vi "STA - Wave V5 Host_Wait.vi"() -> ()   [LabVIEW 2015]
doc: "The continuous acquisition mode tells the FPGA to acquire points indefinitely until a stop command is issued or until an error is encountered (FIFO overflow, module underflow, and so on). \n\nIn this acquisition mode, explicitly call the appropriate rwfm_ConfigTiming VI and set the host application's data buffer to be many times larger than the read size. The examples use a 10X size by default. If the host application's data buffer fills, then the FPGA experiences a FIFO overflow causing the acquisition to stop."
uses:
  <vilib>/rvi/interface/nirviCloseFPGA/nirviCloseFPGA.xnode
  <vilib>/FPGAPlugInAG/Dynamic/niLvFpga_Close_Dynamic.vi
  <vilib>/NI/cRIO Wfm/cRIO Wfm.lvlib
  <vilib>/rvi/interface/nirviMethod/nirviMethod.xnode
  <vilib>/rvi/interface/nirviMethod/StockFPGA_InlinedMethodWaitForSingleIRQ.vi
  <vilib>/FPGAPlugInAG/Dynamic/niLvFpga_WaitOnIrq_Dynamic.vi
  <vilib>/rvi/interface/nirviOpenFPGA/nirviOpenFPGA.xnode
  C:/Program Files (x86)/National Instruments/LabVIEW 2015/ProjectTemplates/Source/cRIOWfm/FPGA/[FPGA] SAR Acq Main.vi
  D/Documents/LabVIEW Data/STA - Waveform V0/FPGA Bitfiles/SARAcqMain_9074.lvbitx
  FPGA Bitfiles/STA-WaveformV6_FPGATarget2_[FPGA]DeltaSigMa_HoNCM4Xd4J8.lvbitx
  FPGA/[FPGA] DeltaSig Main V6_5Mod.vi
  <vilib>/FPGAPlugInAG/cRIO-9112/niLvFpga_Open_cRIO-9112.vi
  <vilib>/rvi/interface/common/dynamic/niFpgaDynamicAddResources.vi
  <vilib>/NI/cRIO Wfm/AcqRead(InterleavedSGLs).vi
  <vilib>/LabVIEW Targets/FPGA/cRIO/shared/nicrio_ModuleControls/nicrio_cRIO-9234_ConfigModeRing.ctl
panel:
  out "error schleife":errorcluster
  out "Time Measure":dbl
  out "data rate (S/s)":u32
  out "Channel Config":T2(array[cluster]) {"Input Configuration" items=["AC Coupled", "DC Coupled", "IEPE AC Coupled"]}
  in  "Samples per Read":i32
  out "file path":path
  out "error out":errorcluster
  in  "stop":bool
  out "Waveform Graph":waveform(sgl)[](graph)
  out "Buffer Backlog":dbl caption="RT Buffer Backlog [%]" format="%#.2g"
  # "Sampling Info"
  # "Channel Info"
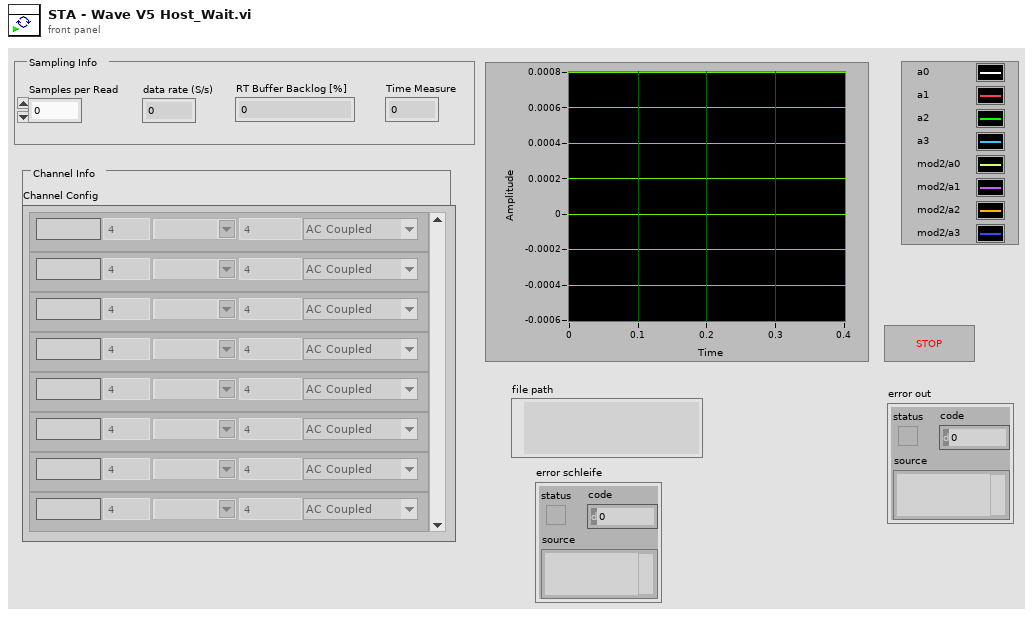
[diagram p1: front panel]
types:
  T1 = typedef "nicrio_cRIO-9234_ConfigModeRing.ctl" = u8
  T2 = cluster{"Channel Name":string, "Sensitivity mV_EU":dbl, "EU":string, "Input Configuration":T1, "dB Ref EU":dbl}[]
  T3 = enum16{"open", "open or create", "create or replace", "create", "open (read-only)"}
  T4 = typedef "Acquisition and Logging Configuration_Waveform.ctl" = cluster{"Data Rate":T5, "Samples per Read":i32, "Number of Reads to Save":i32, "Data File Name":string, "TDMS Properties":T6[], "Number of Channels":i32, "Trigger - RMS Value":dbl, "Trigger - Channel":i32, "Trigger - Time (Minute)":i32, "Channel Config":cluster{"Channel Name":string, "Sensitivity mV_EU":dbl, "EU":string, "Input Configuration":T1, "dB Ref EU":dbl}[], "data rate (S/s)":u32, "Time Measure":dbl}
  T5 = typedef "nicrio_cRIO-9234_DataRatesRing2.ctl" = u8
  T6 = typedef "TDMS Properties.ctl" = cluster{"Name":string, "Value":string}
  T7 = typedef "cRIO Wfm.lvlib/SamplingInfo.ctl" = cluster{"Number of Channels":i32, "Actual Samp Rate":dbl, "Chan Name Array":string[], "EU Chan Array":string[], "dB Ref Chan Array":dbl[]}
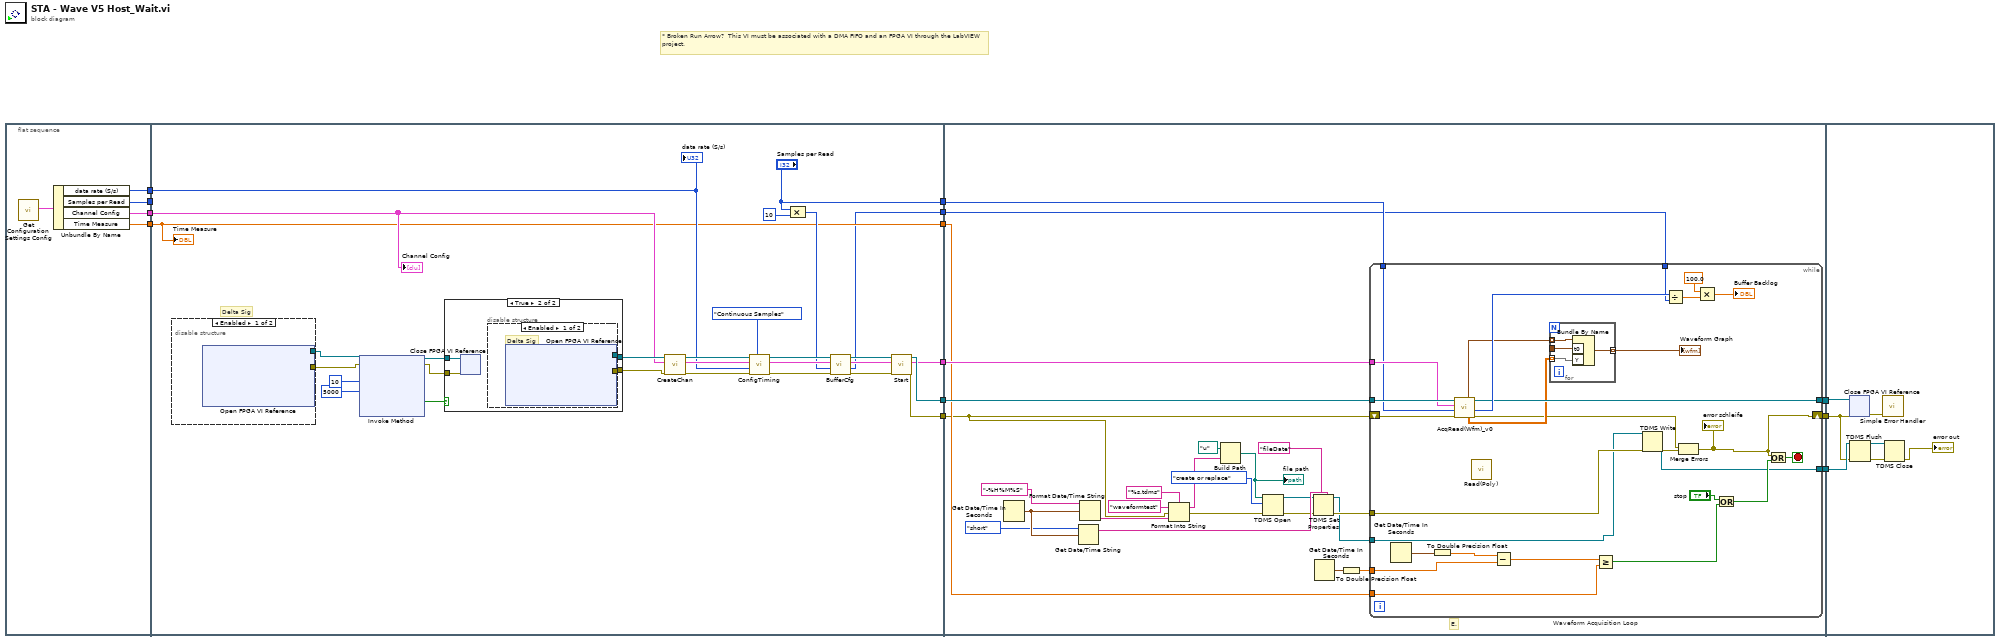
[diagram p0: block diagram]
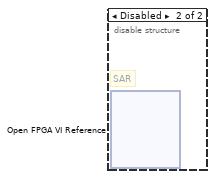
[diagram p2: hidden frame]
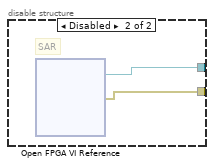
[diagram p4: hidden frame]
diagram:
  # "* Broken Run Arrow?  This VI must be associated with a DMA FIFO and an FPGA VI through the LabVIEW project."
  n1 = flat-sequence {
    tunnel: [w17] -> w13
    tunnel: [w16] -> w12
    tunnel: [w15] -> w11
    tunnel: [w14] -> w10
    tunnel: w13 -> [w28]
    tunnel: w12 -> [_]
    tunnel: w11 -> [w27]
    tunnel: w10 -> [w20]
    tunnel: ["Samples per Read"] -> w9
    tunnel: [w20] -> w8
    tunnel: [w24] -> w7
    tunnel: [w23] -> w6
    tunnel: [w22] -> w5
    tunnel: [w19] -> w4
    tunnel: w9 -> [w64]
    tunnel: w8 -> [w66]
    tunnel: w7 -> [w68]
    tunnel: w6 -> [w67]
    tunnel: w5 -> [w62]
    tunnel: w4 -> [w63]
    tunnel: [w71] -> w3
    tunnel: [w70] -> w2
    tunnel: [w69] -> w1
    tunnel: w3 -> [w125]
    tunnel: w2 -> [w123]
    tunnel: w1 -> [w124]
    frame #0 {
      n2 = call "Get Configuration Settings Config.vi"() -> ("Configuration"=w18:T4)  [unwired: 10 in, 1 out]
      n3 = Unbundle By Name(w18) -> ("data rate (S/s)"=w17:u32, "Samples per Read"=w16:i32, "Channel Config"=w15:T2, "Time Measure"=w14:dbl)
    }
    frame #1 {
      # "Delta Sig"
      n4 = disable-structure shown="Enabled" {
        disable-tunnel: [w49 _] -> w26
        disable-tunnel: [w48 _] -> w25
        frame Enabled {
          n5 = xnode "Open FPGA VI Reference"() -> ("FPGA VI Reference Out"=w49:refnum<k20>, "error out"=w48:errorcluster)  [unwired: 2 in]
        }
        frame Disabled {
          # "SAR"
          n6 = xnode "Open FPGA VI Reference"() -> ("FPGA VI Reference Out"=w51:refnum<k20>, "error out"=w50:errorcluster)  [unwired: 2 in]
        }
      }
      n7 = xnode "Invoke Method"("FPGA VI Reference In"=w26, "error in"=w25, "IRQ Number(s)"=10, "Timeout (ms)"=5000) -> ("FPGA VI Reference Out"=w44:refnum<k20>, "error out"=w45:errorcluster, "Timed Out"=w43:bool)  [unwired: 1 out]
      n8 = case shown="True" w43 {
        tunnel: w44 -> [w53 w57]
        tunnel: w45 -> [w52 w56]
        tunnel: [w53 w55] -> w47
        tunnel: [w52 w54] -> w46
        frame False {
        }
        frame True {
          n9 = xnode "Close FPGA VI Reference"("FPGA VI Reference In"=w57, "error in"=w56) -> ()  [unwired: 1 out]
          n10 = disable-structure shown="Enabled" {
            disable-tunnel: [w59 w61] -> w55
            disable-tunnel: [w58 w60] -> w54
            frame Enabled {
              # "Delta Sig"
              n11 = xnode "Open FPGA VI Reference"() -> ("FPGA VI Reference Out"=w59:refnum<k20>, "error out"=w58:errorcluster)  [unwired: 2 in]
            }
            frame Disabled {
              # "SAR"
              n12 = xnode "Open FPGA VI Reference"() -> ("FPGA VI Reference Out"=w61:refnum<k20>, "error out"=w60:errorcluster)  [unwired: 2 in]
            }
          }
        }
      }
      n13 = call <vilib>:"CreateChan.vi"("Dynamic FPGA Ref"=w47, "Channel Config"=w27, "error in"=w46) -> ("Dynamic FPGA Ref Out"=w34:refnum<k20>, "Sampling Info"=w35:T7, "error out"=w39:errorcluster)  [unwired: 5 in]
      n14 = call <vilib>:"ConfigTiming.vi"("Sample Mode"=enum16{"Finite Samples", "Continuous Samples"}."Continuous Samples", "error in"=w39, "Sample Rate"=w28, "Sampling Info In"=w35, "Dynamic FPGA Ref"=w34) -> ("error out"=w38:errorcluster, "Sampling Info Out"=w37:T7, "Dynamic FPGA Ref Out"=w36:refnum<k20>)  [unwired: 3 in, 1 out]
      n15 = Compound Arithmetic op=MULTIPLY("Samples per Read", 10 ("value")) -> (w32:i32)
      n16 = call <vilib>:"BufferCfg.vi"("error in"=w38, "Buffer Size [Samps per Chan]"=w32, "Sampling Info In"=w37, "Dynamic FPGA Ref"=w36) -> ("error out"=w31:errorcluster, "Buffer Size [Total Samples]"=w19:u32, "Sampling Info Out"=w33:T7, "Dynamic FPGA Ref Out"=w30:refnum<k20>)  [unwired: 4 out]
      n17 = call <vilib>:"Start.vi"("error in"=w31, "Sampling Info In"=w33, "Dynamic FPGA Ref"=w30) -> ("error out"=w22:errorcluster, "Sampling Info Out"=w23:T7, "Dynamic FPGA Ref Out"=w24:refnum<k20>)  [unwired: 6 out]
      "Channel Config" <- w27
      "data rate (S/s)" <- w28
      "Time Measure" <- w20
    }
    frame #2 {
      # "E."
      n18 = Get Date/Time In Seconds() -> (seconds since 1Jan1904=w86:timestamp)
      n19 = Get Date/Time String(date format (0)=enum16{"short", "long", "abbreviated"}."short", seconds (now)=w86) -> (date string=w89:string)  [unwired: 1 in, 1 out]
      n20 = Format Date/Time String(time format string (%c)="-%H%M%S", seconds (now)=w86) -> (date/time string=w76:string)  [unwired: 1 in]
      n21 = Format Into String(format string="%s.tdms", initial string="waveformtest", error in=w62, w76) -> (resulting string=w72:string, error out=w83:errorcluster)
      n22 = Build Path(base path=path "u:/", name or relative path=w72) -> (appended path=w80:path)
      "file path" <- w80
      n23 = TDMS Open(8:w83, 10:T3."create or replace" ("operation (0:open)"), 11:w80) -> (0:w78:errorcluster, 3:w79:refnum<k34>)  [unwired: 4 in]
      n24 = TDMS Set Properties(5:w89, 7:"fileDate" ("property names"), 8:w78, 11:w79) -> (0:w85:errorcluster, 3:w84:refnum<k34>)  [unwired: 2 in, 2 out]
      n25 = Get Date/Time In Seconds() -> (seconds since 1Jan1904=w88:timestamp)
      n26 = To Double Precision Float(number=w88) -> (double precision float=w87:dbl)
      n27 = while "Waveform Acquisition Loop" {
        tunnel: [w112] -> w71
        shift-right: [w90] -> w70
        shift-left: w62 -> [w118]
        tunnel: w84 -> [w94]
        tunnel: w85 -> [w95]
        tunnel: [w93] -> w69
        tunnel: w87 -> [w101]
        tunnel: w66 -> [w100]
        tunnel: w68 -> [w99]
        tunnel: w67 -> [w98]
        tunnel: w64 -> [w97]
        tunnel: w63 -> [w96]
        stop <- w113 stop-if-true
        n28 = Get Date/Time In Seconds() -> (seconds since 1Jan1904=w103:timestamp)
        n29 = To Double Precision Float(number=w103) -> (double precision float=w102:dbl)
        n30 = call <vilib>:"AcqRead(Wfm)_v0.vi"("error in"=w118, "Samps Read per Chan"=w97, "Sampling Info"=w98, "Dynamic FPGA Ref"=w99) -> ("error out"=w108:errorcluster, "Samples Remaining"=w117:u32, "time stamp"=w109:timestamp, "Dynamic FPGA Ref Out"=w112:refnum<k20>, "transposed array"=w110:sgl[][], "Array"=w111:waveform(sgl)[])  [unwired: 2 in]
        n31 = call-poly <vilib>:"Read(Poly).vi"() -> ()  [unwired: 8 in, 4 out]
        n32 = Subtract(x=w102, y=w101) -> (x-y=w104:dbl)
        n33 = for {
          tunnel: w111 -> [w122] mode=indexing
          tunnel: _ -> [w121]
          tunnel: [w120] -> w92 mode=indexing
          tunnel: w110 -> [w119] mode=indexing
          n34 = Bundle By Name(cluster=w122, "t0"=w121, "Y"=w119) -> (w120:waveform(sgl))
        }
        "Waveform Graph" <- w92
        n35 = Greater Or Equal?(x=w104, y=w100) -> (x >= y?=w107:bool)
        n36 = TDMS Write(0:w94, 11:w95) -> (4:w93:refnum<k34>, 15:w91:errorcluster)  [unwired: 4 in, 2 out]
        n37 = Divide(x=w117, y=w96) -> (x/y=w116:dbl)
        n38 = Merge Errors(w108, w91) -> (w90:errorcluster)
        "error schleife" <- w90
        n39 = Multiply(x=100.0, y=w116) -> (x*y=→"Buffer Backlog":dbl)
        n40 = Or(x="stop", y=w107) -> (x .or. y?=w105:bool)
        n41 = Or(x=w90, y=w105) -> (x .or. y?=w113:bool)
      }
    }
    frame #3 {
      n42 = xnode "Close FPGA VI Reference"("FPGA VI Reference In"=w125, "error in"=w123) -> ("error out"=w126:errorcluster)
      n43 = TDMS Flush(4:w123, 7:w124) -> (0:w127:errorcluster, 3:w129:refnum<k34>)
      n44 = call <vilib>:"Simple Error Handler.vi"("error in (no error)"=w126) -> ()  [unwired: 1 in, 8 out]
      n45 = TDMS Close(8:w127, 11:w129) -> (0:→"error out":errorcluster)  [unwired: 1 out]
    }
  }
